vi "PXI-Coerce Rep Rate.vi"(8 "error in (no error)":errorcluster, 9 "AI sampling rate (Hz)":dbl, 10 "AO sampling rate (Hz)":dbl, 11 "Rep rate (Hz)":dbl) -> (0 "error out":errorcluster, 1 "AI npts":i32, 2 "AO npts":i32, 3 "Coerced rep rate (Hz)":dbl)   [LabVIEW 2020]
doc: "Coerces the stimulus repetition rate to prevent relative drifting of input and output. Forces an integer ratio of input and output buffer sizes."
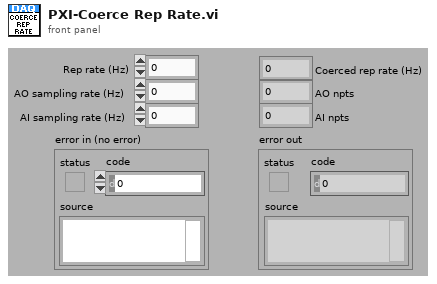
[diagram p1: front panel]
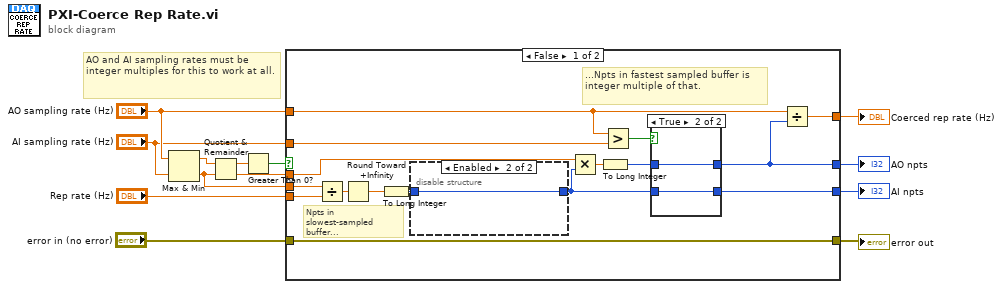
[diagram p0: block diagram]
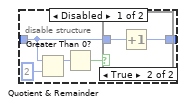
[diagram p2: hidden frame]
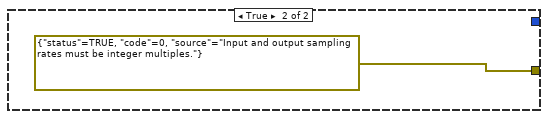
[diagram p5: hidden frame]
diagram:
  # "AO and AI sampling rates must be integer multiples for this to work at all."
  n1 = Max & Min(x="AO sampling rate (Hz)", y="AI sampling rate (Hz)") -> (max(x,y)=w13:dbl, min(x,y)=w8:dbl)
  n2 = Quotient & Remainder(x=w13, y=w8) -> (x-y*floor(x/y)=w12:dbl, floor(x/y)=w6:dbl)
  n3 = Greater Than 0?(x=w12) -> (x > 0?=w11:bool)
  n4 = case shown="False" w11 {
    tunnel: "AO sampling rate (Hz)" -> [w20 _]
    tunnel: "AI sampling rate (Hz)" -> [w24 _]
    tunnel: w8 -> [w29 _]
    tunnel: "Rep rate (Hz)" -> [w28 _]
    tunnel: w6 -> [w26 _]
    tunnel: [w19 _] -> w5
    tunnel: [w21 _] -> w4
    tunnel: [w18 _] -> w3
    tunnel: "error in (no error)" -> [w17 _]
    tunnel: [w17 errorcluster {"status"=TRUE, "code"=0, "source"="Input and output sampling rates must be integer multiples."} ("error out")] -> w1
    frame False {
      # "...Npts in fastest sampled buffer is integer multiple of that."
      # "Npts in slowest-sampled buffer..."
      n5 = Divide(x=w29, y=w28) -> (x/y=w27:dbl)
      n6 = Round Toward +Infinity(x=w27) -> (ceil(x): smallest int >= x=w16:dbl)
      n7 = To Long Integer(number=w16) -> (32bit integer=w15:i32)
      n8 = disable-structure shown="Enabled" {
        disable-tunnel: w15 -> [w31 w38]
        disable-tunnel: [w30 w38] -> w14
        frame Disabled {
          n9 = Quotient & Remainder(x=w31, y=2) -> (x-y*floor(x/y)=w33:i32)  [unwired: 1 out]
          n10 = Greater Than 0?(x=w33) -> (x > 0?=w32:bool)
          n11 = case shown="True" w32 {
            tunnel: [w35 w36] -> w30
            tunnel: w31 -> [w35 w37]
            frame False {
            }
            frame True {
              n12 = Increment(x=w37) -> (x+1=w36:i32)
            }
          }
        }
        frame Enabled {
        }
      }
      n13 = Multiply(x=w26, y=w14) -> (x*y=w25:dbl)
      n14 = To Long Integer(number=w25) -> (32bit integer=w22:i32)
      n15 = Greater?(x=w20, y=w24) -> (0:w23:bool)
      n16 = case shown="True" w23 {
        tunnel: w22 -> [w40 w42]
        tunnel: [w39 w42] -> w19
        tunnel: w14 -> [w39 w41]
        tunnel: [w40 w41] -> w21
        frame False {
        }
        frame True {
        }
      }
      n17 = Divide(x=w20, y=w19) -> (x/y=w18:dbl)
    }
    frame True {
    }
  }
  "error out" <- w1
  "AO npts" <- w5
  "AI npts" <- w4
  "Coerced rep rate (Hz)" <- w3
